vi "ReadCommand-SubVI.vi"(3 "handle":i32, 4 "Motion #":u32, 5 "Enable\n(True)":bool) -> (0 "Enable Move\n(TRUE)":bool, 1 "Direction":dbl, 2 "Axis":enum16{"X", "Y", "Z"}(ring))   [LabVIEW 2014]
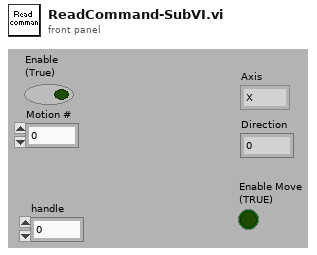
[diagram p1: front panel]
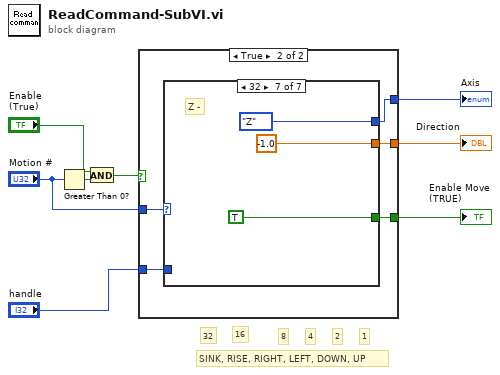
[diagram p0: block diagram]
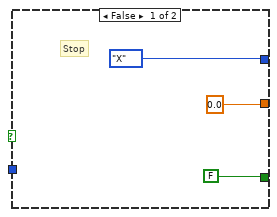
[diagram p2: hidden frame]
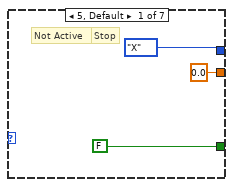
[diagram p3: hidden frame]
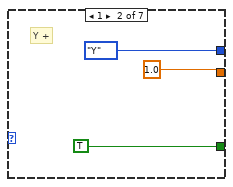
[diagram p4: hidden frame]
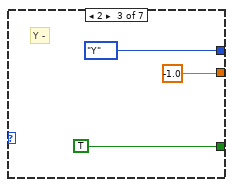
[diagram p5: hidden frame]
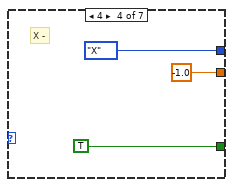
[diagram p6: hidden frame]
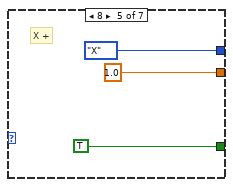
[diagram p7: hidden frame]
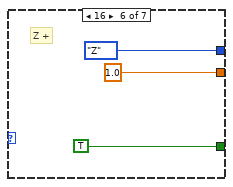
[diagram p8: hidden frame]
diagram:
  # "32"
  # "16"
  # "8"
  # "4"
  # "2"
  # "1"
  # "SINK, RISE, RIGHT, LEFT, DOWN, UP"
  n1 = Greater Than 0?(x="Motion #") -> (x > 0?=w8:bool)
  n2 = And(x="Enable\n(True)", y=w8) -> (x .and. y?=w7:bool)
  n3 = case shown="True" w7 {
    tunnel: [FALSE w16] -> w1
    tunnel: [enum16{"X", "Y"}."X" ("Axis 2") w15] -> w3
    tunnel: "handle" -> [_ w14]
    tunnel: "Motion #" -> [_ w13]
    tunnel: [0.0 ("Move size (mm)") w12] -> w2
    frame False {
      # "Stop"
    }
    frame True {
      n4 = case shown="32" w13 {
        tunnel: w14 -> [_ _ _ _ _ _ _]
        tunnel: [FALSE TRUE TRUE TRUE TRUE TRUE TRUE] -> w16
        tunnel: [enum16{"X", "Y"}."X" ("Axis 2") enum16{"X", "Y"}."Y" ("Axis 2") enum16{"X", "Y"}."Y" ("Axis 2") enum16{"X", "Y"}."X" ("Axis 2") enum16{"X", "Y"}."X" ("Axis 2") enum16{"X", "Y", "Z"}."Z" ("Axis 2") enum16{"X", "Y", "Z"}."Z" ("Axis 2")] -> w15
        tunnel: [0.0 ("Move size (mm)") 1.0 ("Move size (mm)") -1.0 ("Move size (mm)") -1.0 ("Move size (mm)") 1.0 ("Move size (mm)") 1.0 ("Move size (mm)") -1.0 ("Move size (mm)")] -> w12
        frame 5, Default {
          # "Stop"
          # "Not Active"
        }
        frame 1 {
          # "Y +"
        }
        frame 2 {
          # "Y -"
        }
        frame 4 {
          # "X -"
        }
        frame 8 {
          # "X +"
        }
        frame 16 {
          # "Z +"
        }
        frame 32 {
          # "Z -"
        }
      }
    }
  }
  "Axis" <- w3
  "Direction" <- w2
  "Enable Move\n(TRUE)" <- w1
